vi "Queue_Driver.vi"(0 "Queue Name":string, 5 "Enqueue State":string, 7 "Array of States":string[](array[string]), 11 "error in (no error)":errorcluster, 13 "Queue Operation":T1=enum."Enqueue N Element") -> (4 "Dequeued State":string, 15 "error out":errorcluster)   [LabVIEW 2020]
uses:
  Typedefs/Queue_Operations.ctl
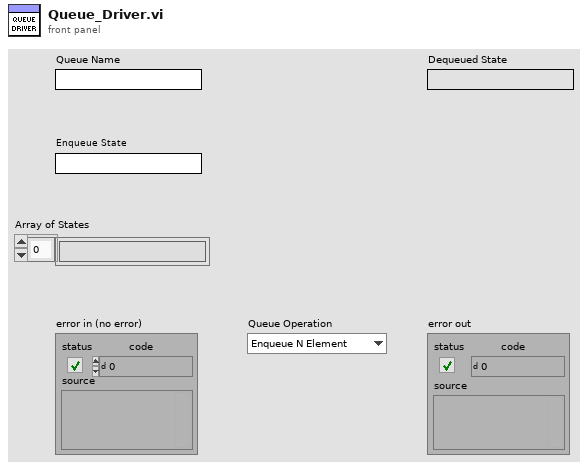
[diagram p1: front panel]
types:
  T1 = typedef "Queue_Operations.ctl" = enum16{"Obtain Queue", "Enqueue", "Enqueue N Element", "Enqueue at First", "Dequeue", "Release Queue", "Queue Status", "Flush Queue"}
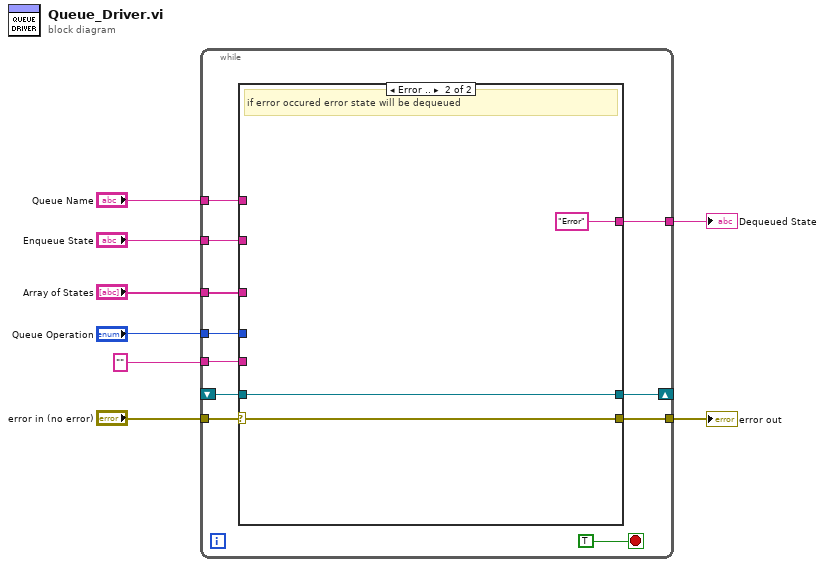
[diagram p0: block diagram]
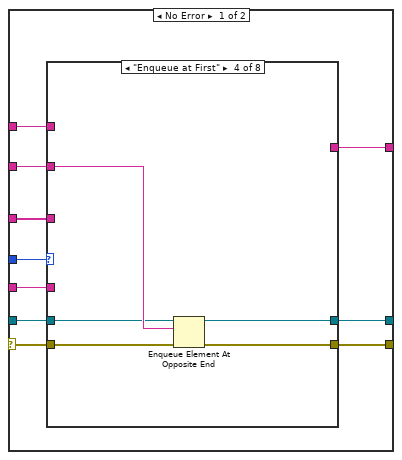
[diagram p2: hidden frame]
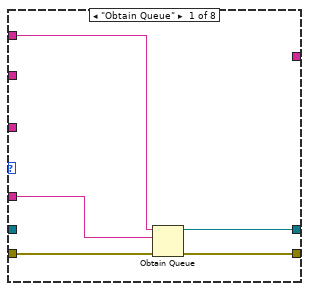
[diagram p3: hidden frame]
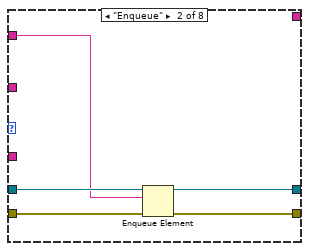
[diagram p4: hidden frame]
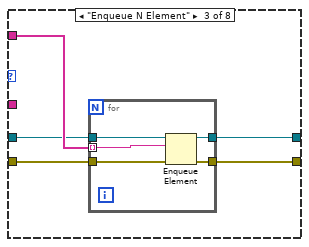
[diagram p5: hidden frame]
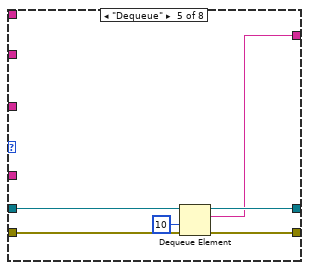
[diagram p6: hidden frame]
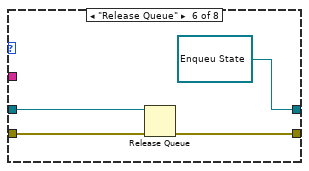
[diagram p7: hidden frame]
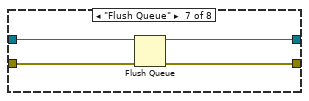
[diagram p8: hidden frame]
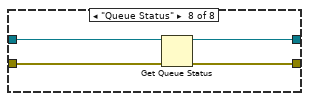
[diagram p9: hidden frame]
diagram:
  n1 = while {
    tunnel: "Queue Operation" -> [w19]
    tunnel: "Enqueue State" -> [w18]
    tunnel: "Array of States" -> [w17]
    tunnel: "Queue Name" -> [w16]
    tunnel: "error in (no error)" -> [w15]
    tunnel: [w14] -> w4
    shift-right: [w13] -> _
    shift-left: _ -> [w12]
    tunnel: [w11] -> w3
    tunnel: "" ("Enqueue State") -> [w9]
    stop <- TRUE stop-if-true
    n2 = case shown="Error .." w15 {
      selector: w15 -> [w25 w74]
      tunnel: w19 -> [w29 _]
      tunnel: w18 -> [w28 _]
      tunnel: w17 -> [w27 _]
      tunnel: w16 -> [w26 _]
      tunnel: [w24 w74] -> w14
      tunnel: [w23 w75] -> w13
      tunnel: w12 -> [w22 w75]
      tunnel: [w21 "Error" ("Enqueu State")] -> w11
      tunnel: w9 -> [w20 _]
      frame No Error {
        n3 = case shown="\"Enqueue at First\"" w29 {
          tunnel: w28 -> [_ w36 _ w52 _ _ _ _]
          tunnel: w27 -> [_ _ w42 _ _ _ _ _]
          tunnel: w26 -> [w32 _ _ _ _ _ _ _]
          tunnel: w25 -> [w34 w39 w44 w54 w60 w64 w68 w72]
          tunnel: [w33 w38 w43 w53 w59 w63 w67 w71] -> w24
          tunnel: [w31 w35 w40 w50 w57 refnum<queue> refnum ("queue out") w66 w69] -> w23
          tunnel: w22 -> [_ w37 w41 w51 w58 w62 w65 w70]
          tunnel: [_ _ _ _ w56 _ _ _] -> w21
          tunnel: w20 -> [w30 _ _ _ _ _ _ _]
          frame "Obtain Queue" {
            n4 = Obtain Queue(name (unnamed)=w32, element data type=w30, error in (no error)=w34) -> (queue out=w31:refnum<queue>, error out=w33:errorcluster)  [unwired: 2 in, 1 out]
          }
          frame "Enqueue" {
            n5 = Enqueue Element(queue=w37, element=w36, error in (no error)=w39) -> (queue out=w35:refnum<queue>, error out=w38:errorcluster)  [unwired: 1 in, 1 out]
          }
          frame "Enqueue N Element" {
            n6 = for {
              tunnel: w44 -> [w49]
              tunnel: [w48] -> w43
              tunnel: w42 -> [w47] mode=indexing
              tunnel: w41 -> [w46]
              tunnel: [w45] -> w40
              n7 = Enqueue Element(queue=w46, element=w47, error in (no error)=w49) -> (queue out=w45:refnum<queue>, error out=w48:errorcluster)  [unwired: 1 in, 1 out]
            }
          }
          frame "Enqueue at First" {
            n8 = Enqueue Element At Opposite End(queue=w51, element=w52, error in (no error)=w54) -> (queue out=w50:refnum<queue>, error out=w53:errorcluster)  [unwired: 1 in, 1 out]
          }
          frame "Dequeue" {
            n9 = Dequeue Element(queue=w58, timeout in ms (-1)=10, error in (no error)=w60) -> (queue out=w57:refnum<queue>, element=w56:string, error out=w59:errorcluster)  [unwired: 1 out]
          }
          frame "Release Queue" {
            n10 = Release Queue(queue=w62, error in (no error)=w64) -> (error out=w63:errorcluster)  [unwired: 1 in, 2 out]
          }
          frame "Flush Queue" {
            n11 = Flush Queue(queue=w65, error in (no error)=w68) -> (queue out=w66:refnum<queue>, error out=w67:errorcluster)  [unwired: 1 out]
          }
          frame "Queue Status" {
            n12 = Get Queue Status(queue=w70, error in (no error)=w72) -> (queue out=w69:refnum<queue>, error out=w71:errorcluster)  [unwired: 1 in, 6 out]
          }
        }
      }
      frame Error {
        # "if error occured error state will be dequeued"
      }
    }
  }
  "error out" <- w4
  "Dequeued State" <- w3
